vi "closeListener.vi"(8 "error in (no error)":errorcluster, 9 "close":bool, 10 "actions":enum16{"read", "write"}(ring), 11 "NetworkServer in":refnum<class "NetworkServer.lvclass">) -> (0 "error out":errorcluster, 1 "close":bool, 3 "NetworkServer out":refnum<class "NetworkServer.lvclass">)   [LabVIEW 2011, in "Hardware.lvlib" / "HWControllers.lvlib" / "NetworkServer.lvclass"]
uses:
  NetworkServer.lvclass
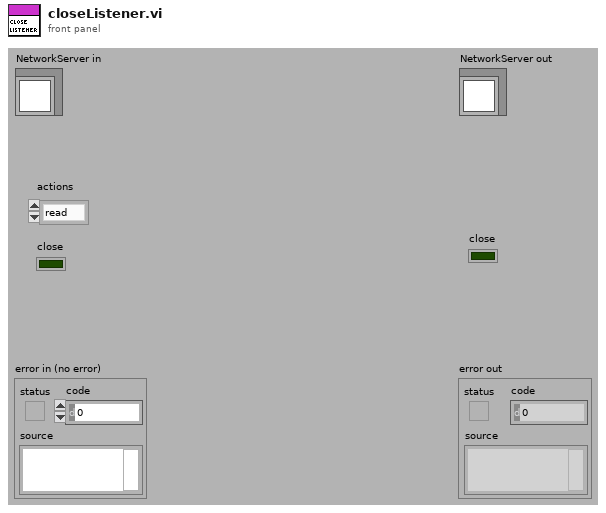
[diagram p1: front panel]
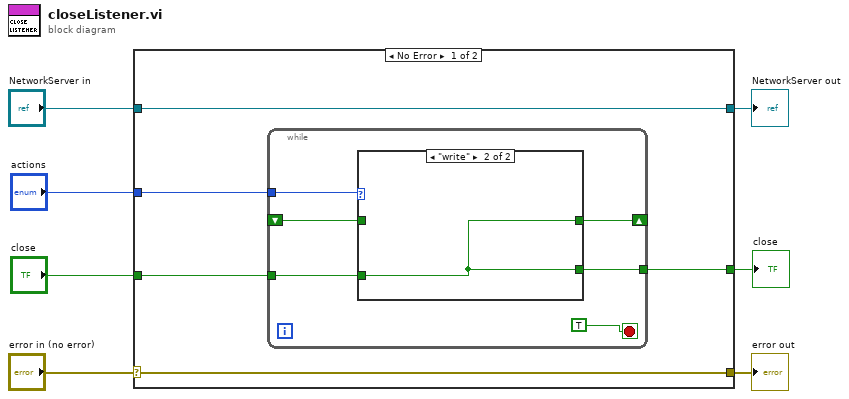
[diagram p0: block diagram]
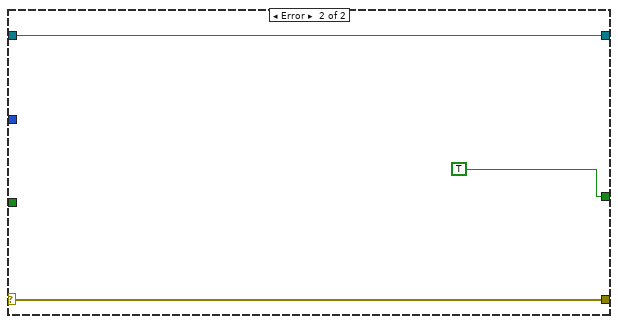
[diagram p3: hidden frame]
diagram:
  n1 = case shown="No Error" "error in (no error)" {
    selector: "error in (no error)" -> [w11 w23]
    tunnel: [w11 w23] -> w6
    tunnel: [w12 w22] -> w4
    tunnel: "NetworkServer in" -> [w12 w22]
    tunnel: "actions" -> [w10 _]
    tunnel: "close" -> [w9 _]
    tunnel: [w8 TRUE] -> w1
    frame No Error {
      n2 = while {
        tunnel: w10 -> [w18]
        tunnel: w9 -> [w17]
        shift-right: [w16] -> _
        shift-left: _ -> [w15]
        tunnel: [w14] -> w8
        stop <- TRUE stop-if-true
        n3 = case shown="\"write\"" w18 {
          tunnel: w17 -> [_ w20]
          tunnel: [w19 w20] -> w16
          tunnel: w15 -> [w19 _]
          tunnel: [w19 w20] -> w14
          frame "read", Default {
          }
          frame "write" {
          }
        }
      }
    }
    frame Error {
    }
  }
  "error out" <- w6
  "NetworkServer out" <- w4
  "close" <- w1
